vi "Read Low Resolution Video.vi"(8 "error in (no error)":errorcluster, 11 "input cluster":T4) -> (0 "error out":errorcluster, 3 "RGB image":picture)   [LabVIEW 2013]
uses:
  Video Resolution Control.ctl
  Video Format Control.ctl
  Depth Resolution Control.ctl
  <vilib>/picture/picture.llb/Draw True-Color Pixmap.vi
  libkinect_wrapper.dll
panel:
  out "raw video data":u16[](array[numeric])
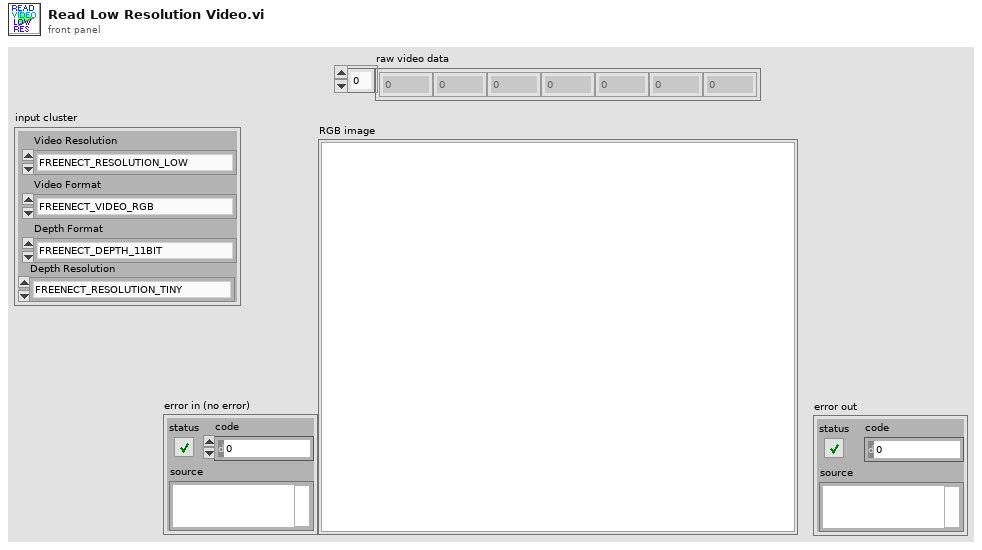
[diagram p1: front panel]
types:
  T1 = typedef "Video Resolution Control.ctl" = enum32{"FREENECT_RESOLUTION_LOW", "FREENECT_RESOLUTION_MEDIUM", "FREENECT_RESOLUTION_HIGH"}
  T2 = typedef "Video Format Control.ctl" = enum32{"FREENECT_VIDEO_RGB", "FREENECT_VIDEO_BAYER", "FREENECT_VIDEO_IR_8BIT", "FREENECT_VIDEO_IR_10BIT", "FREENECT_VIDEO_IR_10BIT_PACKED", "FREENECT_VIDEO_YUV_RGB", "FREENECT_VIDEO_YUV_RAW"}
  T3 = typedef "Depth Resolution Control.ctl" = enum16{"FREENECT_RESOLUTION_TINY", "FREENECT_RESOLUTION_LOW", "FREENECT_RESOLUTION_MEDIUM"}
  T4 = cluster{"Video Resolution":T1, "Video Format":T2, "Depth Format":enum32{"FREENECT_DEPTH_11BIT", "FREENECT_DEPTH_10BIT", "FREENECT_DEPTH_11BIT_PACKED", "FREENECT_DEPTH_10BIT_PACKED", "FREENECT_DEPTH_REGISTERED", "FREENECT_DEPTH_MM"}, "Depth Resolution":T3}
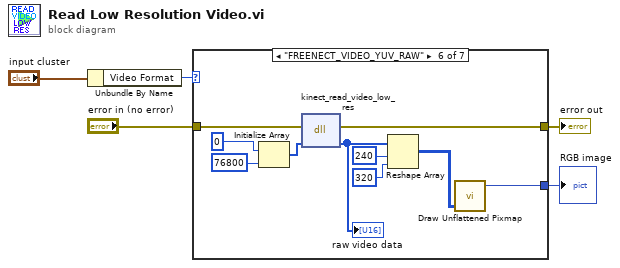
[diagram p0: block diagram]
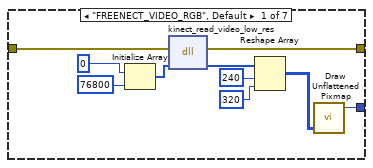
[diagram p2: hidden frame]
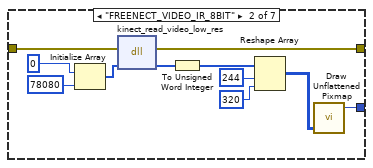
[diagram p3: hidden frame]
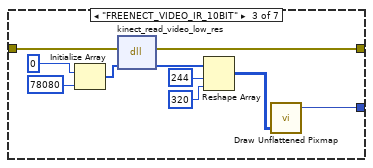
[diagram p4: hidden frame]
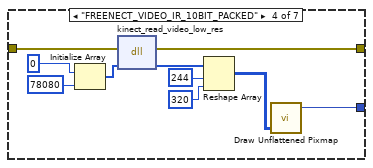
[diagram p5: hidden frame]
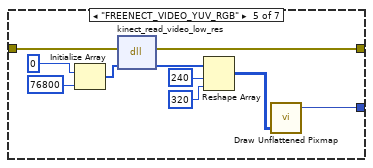
[diagram p6: hidden frame]
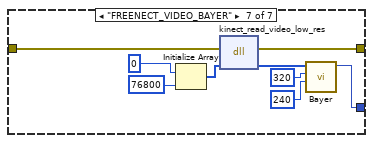
[diagram p7: hidden frame]
diagram:
  n1 = Unbundle By Name("input cluster") -> ("Video Format"=w4:T2)
  n2 = case shown="\"FREENECT_VIDEO_YUV_RAW\"" w4 {
    tunnel: [w8 w16 w28 w38 w48 w58 w67] -> w3
    tunnel: [w7 w19 w29 w39 w49 w59 w71] -> w2
    tunnel: "error in (no error)" -> [w6 w20 w30 w40 w50 w60 w72]
    frame "FREENECT_VIDEO_RGB", Default {
      n3 = Initialize Array(u32 0 ("U32"), 76800 ("dimension size")) -> (w14:u32[])
      n4 = dll-call lib="libkinect_wrapper.*" fn="kinect_read_video_low_res"(error in=w6, "video"=w14) -> (error out=w7:errorcluster, "video"=w12:u32[])  [unwired: 3 in, 1 out]
      n5 = Reshape Array(w12, 240, 320) -> (w11:u32[][])
      n6 = call-poly <vilib>:"Draw Unflattened Pixmap.vi"("data (RGB format)"=w11) -> ("new picture"=w8:picture)  [unwired: 8 in]
    }
    frame "FREENECT_VIDEO_IR_8BIT" {
      n7 = Initialize Array(u8 0 ("U32"), 78080 ("dimension size")) -> (w25:u8[])
      n8 = dll-call lib="libkinect_wrapper.*" fn="kinect_read_video_low_res"(error in=w20, "video"=w25) -> (error out=w19:errorcluster, "video"=w18:u8[])  [unwired: 3 in, 1 out]
      n9 = To Unsigned Word Integer(number=w18) -> (unsigned 16bit integer=w17:u16[])
      n10 = Reshape Array(w17, 244, 320) -> (w23:u16[][])
      n11 = call-poly <vilib>:"Draw Unflattened Pixmap.vi"("data (RGB format)"=w23) -> ("new picture"=w16:picture)  [unwired: 8 in]
    }
    frame "FREENECT_VIDEO_IR_10BIT" {
      n12 = Initialize Array(u16 0 ("U32"), 78080 ("dimension size")) -> (w35:u16[])
      n13 = dll-call lib="libkinect_wrapper.*" fn="kinect_read_video_low_res"(error in=w30, "video"=w35) -> (error out=w29:errorcluster, "video"=w27:u16[])  [unwired: 3 in, 1 out]
      n14 = Reshape Array(w27, 244, 320) -> (w33:u16[][])
      n15 = call-poly <vilib>:"Draw Unflattened Pixmap.vi"("data (RGB format)"=w33) -> ("new picture"=w28:picture)  [unwired: 8 in]
    }
    frame "FREENECT_VIDEO_IR_10BIT_PACKED" {
      n16 = Initialize Array(u16 0 ("U32"), 78080 ("dimension size")) -> (w45:u16[])
      n17 = dll-call lib="libkinect_wrapper.*" fn="kinect_read_video_low_res"(error in=w40, "video"=w45) -> (error out=w39:errorcluster, "video"=w37:u16[])  [unwired: 3 in, 1 out]
      n18 = Reshape Array(w37, 244, 320) -> (w43:u16[][])
      n19 = call-poly <vilib>:"Draw Unflattened Pixmap.vi"("data (RGB format)"=w43) -> ("new picture"=w38:picture)  [unwired: 8 in]
    }
    frame "FREENECT_VIDEO_YUV_RGB" {
      n20 = Initialize Array(u32 0 ("U32"), 76800 ("dimension size")) -> (w55:u32[])
      n21 = dll-call lib="libkinect_wrapper.*" fn="kinect_read_video_low_res"(error in=w50, "video"=w55) -> (error out=w49:errorcluster, "video"=w47:u32[])  [unwired: 3 in, 1 out]
      n22 = Reshape Array(w47, 240, 320) -> (w53:u32[][])
      n23 = call-poly <vilib>:"Draw Unflattened Pixmap.vi"("data (RGB format)"=w53) -> ("new picture"=w48:picture)  [unwired: 8 in]
    }
    frame "FREENECT_VIDEO_YUV_RAW" {
      n24 = Initialize Array(u16 0 ("U32"), 76800 ("dimension size")) -> (w65:u16[])
      n25 = dll-call lib="libkinect_wrapper.*" fn="kinect_read_video_low_res"(error in=w60, "video"=w65) -> (error out=w59:errorcluster, "video"=w57:u16[])  [unwired: 3 in, 1 out]
      "raw video data" <- w57
      n26 = Reshape Array(w57, 240, 320) -> (w63:u16[][])
      n27 = call-poly <vilib>:"Draw Unflattened Pixmap.vi"("data (RGB format)"=w63) -> ("new picture"=w58:picture)  [unwired: 8 in]
    }
    frame "FREENECT_VIDEO_BAYER" {
      n28 = Initialize Array(u8 0, 76800 ("dimension size")) -> (w74:u8[])
      n29 = dll-call lib="libkinect_wrapper.*" fn="kinect_read_video_low_res"(error in=w72, "video"=w74) -> (error out=w71:errorcluster, "video"=w70:u8[])  [unwired: 3 in, 1 out]
      n30 = call "Bayer.vi"("Height"=240, "Width"=320, "Array"=w70) -> ("new picture"=w67:picture)  [unwired: 8 in]
    }
  }
  "RGB image" <- w3
  "error out" <- w2
